vi "PMT_plus_Kiethley2450_plus_rotationstage.vi"() -> ()   [LabVIEW 2022 SP3]
uses:
  <vilib>/Analysis/1siggen.llb/Ramp Pattern by Delta.vi
  <vilib>/Utility/file.llb/Write Delimited Spreadsheet (string).vi
  <vilib>/Utility/file.llb/Write Delimited Spreadsheet (DBL).vi
  <vilib>/Analysis/NI_AALBase.lvlib
  C:/Users/Public/OneDrive/Desktop/test_save_lv22/Close.vi/Close Folder/Users/Public/OneDrive/Desktop/Keithley_2450_2470_1_4_0_LV2015_NewReadme2_2450-LV2015-1.4.0/Keithley 2450/Keithley 2450.lvlib
  C:/Users/Public/OneDrive/Desktop/PMT program/SampleCodeLabView/Kinesis_with_LabVIEW_Examples_LV12 - v3/Thorlabs.MotionControl.Controls.dll
  C:/Users/Public/OneDrive/Desktop/PMT program/SampleCodeLabView/Kinesis_with_LabVIEW_Examples_LV12 - v3/ThorLabs.MotionControl.KCube.DCServoCLI.dll
panel:
  in  "wait for move (ms)":u32=2000
  out "PC":dbl caption="Current Rotation Position"
  in  "quarter waveplate p2":dbl=221.0 format="%#_13g"
  in  "quarter waveplate p1":dbl=131.0 format="%#_13g"
  in  "Motor Controller\nSerialNumber":string="27268499"
  in  "KCubeDCServoControl":refnum<k24>(container)
  in  "Loop?":bool
  out "error out":errorcluster
  out "current 2450":dbl=2.5622937e-12 format="%e"
  out "Serial Configuration":T1={"Baud Rate"=9600, "Parity"=0, "Data Bits"=8, "Stop Bits"=10, "Flow Control"=0} {"Flow Control" items=["None", "XON/XOFF", "RTS/CTS", "XON/XOFF & RTS/CTS", "DTR/DSR", "XON/XOFF & DTR/DSR"]; "Stop Bits" items=["1.0"=10, "1.5"=15, "2.0"=20]; "Data Bits" items=["7"=7, "8"=8]; "Parity" items=["None", "Odd", "Even", "Mark", "Space"]; "Baud Rate" items=["300"=300, "600"=600, "1200"=1200, "2400"=2400, "4800"=4800, "9600"=9600, "19200"=19200]}
  in  "Use PMT?":bool=TRUE
  out "XY Graph":cluster{dbl[], dbl[]}(graph)={[-1.0, -0.5, 0.0], [45.5, 47.5, 49.0]}
  out "Actual Voltage 2450":dbl
  in  "Num Current Meas":i32=20
  in  "Path":path=path "C:/Users/Public/OneDrive/Desktop/test.txt"
  in  "error in (no error)":errorcluster
  in  "VISA resource name":refnum<visa-resource-name>="GPIB0::1::INSTR"
  out "Set Voltage 2450":dbl
  in  "Step Size (V)":dbl=0.5 format="%#_13g"
  in  "End V":dbl=-1.0 format="%#_13g"
  in  "Start V":dbl format="%#_13g"
  in  "Source Limit Level (0.1)":dbl=1e-08
  out "standard deviation":dbl
  out "mean":dbl=49.0
  out "data":u32[](array[numeric])=[49, 49]
  out "OLD":bool
  out "DB":u32[](array[numeric])=[49, 0, 0, 0, 0, 0, 0, 0, 0, 0, 0, 0, 0, 0, 0, 0]
  out "Overload":i32
  out "Gate Number":i32=1
  in  "Correction":bool=TRUE
  out "Num Gates Read":i32=2
  out "Gate Time Read":i32=100 caption="Gate time Read"
  out "Num Gates Set":i32=2
  out "Gate Time Set":i32=100
  out "PowerD":i32 caption="Power\nRead Data"
  out "Handle Number":i32=173123648
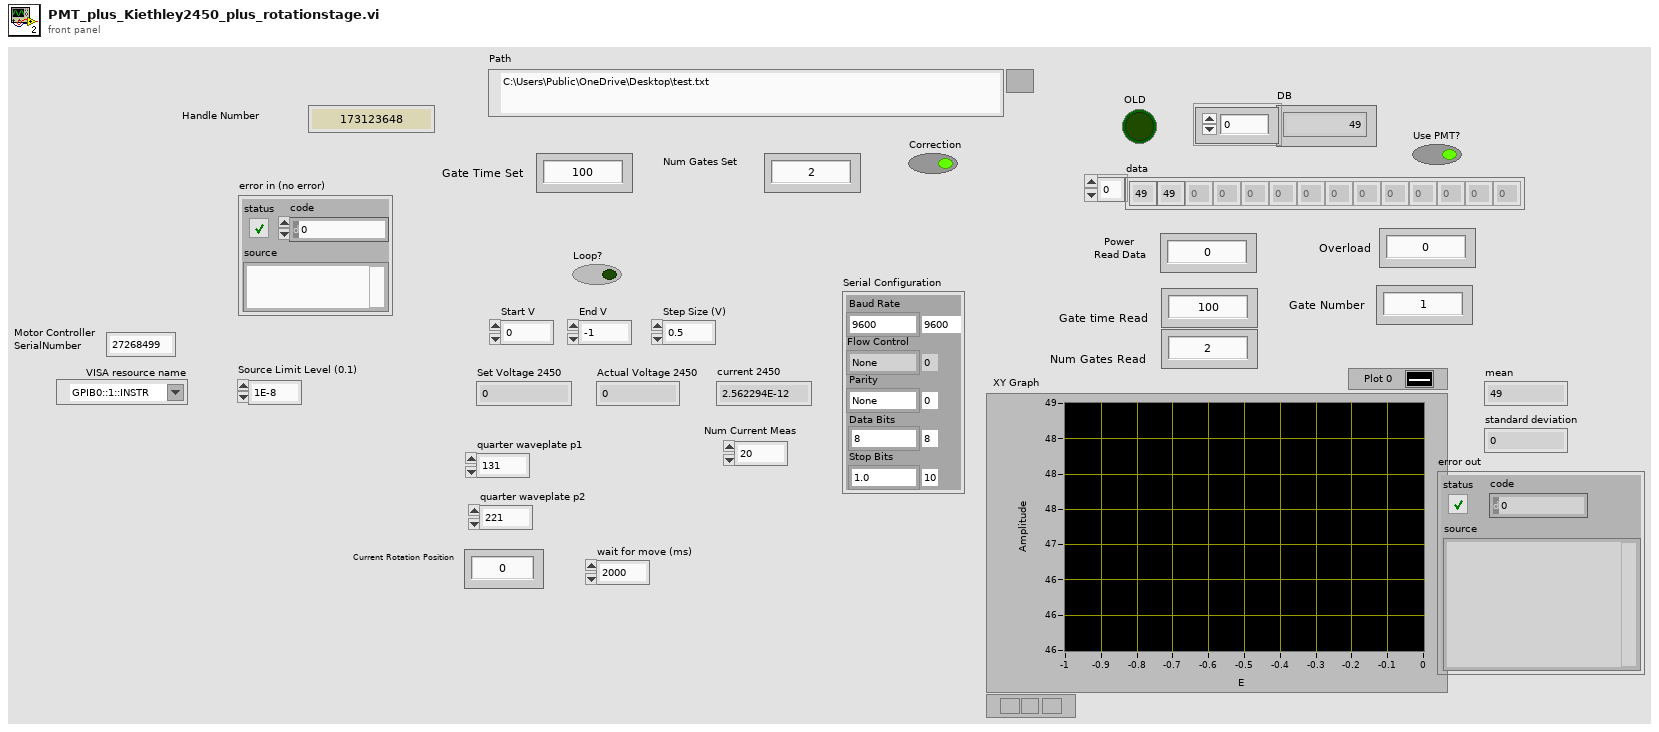
[diagram p1: front panel]
types:
  T1 = cluster{"Baud Rate":u32, "Parity":u16, "Data Bits":u16, "Stop Bits":u16, "Flow Control":u16}
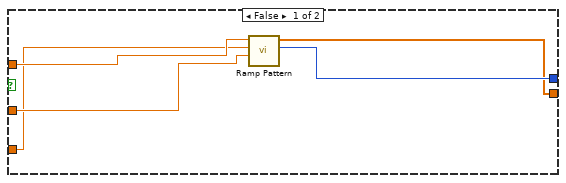
[diagram p2: hidden frame]
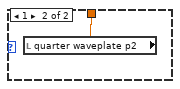
[diagram p3: hidden frame]
diagram:
  n1 = flat-sequence {
    tunnel: [w46] -> w20
    tunnel: [w37] -> w19
    tunnel: ["Path"] -> w18
    tunnel: [w36] -> w17
    tunnel: [w25] -> w16
    tunnel: [w22] -> w1
    tunnel: w20 -> [w82]
    tunnel: [w82] -> w15
    tunnel: w19 -> [w81]
    tunnel: [w81] -> w13
    tunnel: w18 -> [w80]
    tunnel: [w80] -> w11
    tunnel: w17 -> [w79]
    tunnel: [w79] -> w9
    tunnel: [w78] -> w7
    tunnel: w16 -> [w78]
    tunnel: ["wait for move (ms)"] -> w4
    tunnel: [w76] -> w2
    tunnel: w1 -> [w76]
    tunnel: w15 -> [w93]
    tunnel: [w93] -> w14
    tunnel: w13 -> [w92]
    tunnel: [w92] -> w12
    tunnel: w11 -> [w91]
    tunnel: [w91] -> w10
    tunnel: w9 -> [w90]
    tunnel: [w90] -> w8
    tunnel: w7 -> [w89]
    tunnel: [w88] -> w6
    tunnel: [w84] -> w5
    tunnel: w4 -> [w84]
    tunnel: [w83] -> w3
    tunnel: w2 -> [w83]
    tunnel: w14 -> [w105]
    tunnel: w12 -> [w104]
    tunnel: [w103] -> w21
    tunnel: w10 -> [w102]
    tunnel: w8 -> [w97]
    tunnel: w6 -> [w96]
    tunnel: w5 -> [w95]
    tunnel: w3 -> [w94]
    tunnel: w21 -> [w570]
    frame #0 {
      # "open PMT and turn on power"
      n2 = local write "quarter waveplate p2"("quarter waveplate p2") -> ()
      n3 = local write "quarter waveplate p1"("quarter waveplate p1") -> ()
      n4 = call "Open.vi"("Serial Number"="30430219") -> ("Handle Number"=w50:i32)  [unwired: 9 in, 1 out]
      "Handle Number" <- w50
      n5 = case shown="True" "Loop?" {
        tunnel: "Start V" -> [w57 w68]
        tunnel: "End V" -> [w56 w66]
        tunnel: [w59 w65] -> w36
        tunnel: [w60 w64] -> w37
        tunnel: "Step Size (V)" -> [w58 w62]
        frame False {
          n6 = call-poly <vilib>:"Ramp Pattern.vi"("start"=w57, "end"=w56, "delta"=w58) -> ("samples"=w60:i32, "Ramp Pattern"=w59:dbl[])  [unwired: 6 in, 1 out]
        }
        frame True {
          w63 = -1.0
          n7 = Multiply(x=w62, y=w63) -> (x*y=w61:dbl)
          n8 = Multiply(x=w66, y=w63) -> (x*y=w67:dbl)
          n9 = call-poly <vilib>:"Ramp Pattern.vi"("start"=w68, "end"=w66, "delta"=w62) -> ("samples"=w72:i32, "Ramp Pattern"=w69:dbl[])  [unwired: 6 in, 1 out]
          n10 = call-poly <vilib>:"Ramp Pattern.vi"("start"=w67, "end"=w68, "delta"=w62) -> ("samples"=w75:i32, "Ramp Pattern"=w71:dbl[])  [unwired: 6 in, 1 out]
          n11 = call-poly <vilib>:"Ramp Pattern.vi"("start"=w66, "end"=w67, "delta"=w61) -> ("samples"=w73:i32, "Ramp Pattern"=w70:dbl[])  [unwired: 6 in, 1 out]
          n12 = Add(x=w72, y=w73) -> (x+y=w74:i32)
          n13 = Build Array (concatenate)(w69, w70, w71) -> (w65:dbl[])
          n14 = Add(x=w74, y=w75) -> (x+y=w64:i32)
        }
      }
      n15 = call "Read HV.vi"("handle"=w50) -> ("HV out"=w49:i32, "handle out"=w53:i32)  [unwired: 8 in, 1 out]
      n16 = Boolean To (0,1)(Boolean="Use PMT?") -> (0, 1=w51:i16)
      n17 = local write "PowerD"(w49) -> ()
      n18 = To Long Integer(number=w51) -> (32bit integer=w52:i32)
      n19 = call "Set HV.vi"("HV"=w52, "handle"=w53) -> ("handle out"=w55:i32)  [unwired: 8 in, 1 out]
      n20 = property class="KCubeDCServoControl"(reference="KCubeDCServoControl", "SerialNumber"="Motor Controller\nSerialNumber") -> (reference out=w35:refnum<k24>)  [unwired: 1 in, 1 out]
      n21 = invoke class="KCubeDCServoControl" method="CreateDevice"(reference=w35) -> (reference out=w32:refnum<k24>)  [unwired: 2 in, 2 out]
      n22 = property class="KCubeDCServoControl"(reference=w32) -> ("Device"=w22:refnum<k24>)  [unwired: 1 in, 2 out]
      n23 = call "Read HV.vi"("handle"=w55) -> ("HV out"=w54:i32, "handle out"=w46:i32)  [unwired: 8 in, 1 out]
      n24 = local write "PowerD"(w54) -> ()
      n25 = invoke class="KCubeDCServo" method="GetPositionCounter"(reference=w22) -> (reference out=w28:refnum<k24>, "GetPositionCounter"=w31:i32)  [unwired: 2 in, 1 out]
      n26 = Divide(x=w31, y=1919.6418578623338) -> (x/y=w29:dbl)
      n27 = local write "PC"(w29) -> ()
      n28 = invoke class="KCubeDCServo" method="SetMoveAbsolutePosition"(reference=w28, "position"="quarter waveplate p1") -> (reference out=w27:refnum<k24>)  [unwired: 2 in, 3 out]
      n29 = invoke class="KCubeDCServo" method="MoveAbsolute"(reference=w27, "waitTimeout"=0) -> (reference out=w25:refnum<k24>)  [unwired: 2 in, 3 out]
      n30 = Build Array("# SetVoltage2450(V) ActualVoltage2450(V) CountsMean CountsStd Current2450(uA) Current2450Std(uA)") -> (w41:string[])
      n31 = call-poly <vilib>:"Write Delimited Spreadsheet.vi"("file path (dialog if empty)"="Path", "1D data"=w41, "append to file? (new file:F)"=TRUE) -> ()  [unwired: 11 in, 2 out]
    }
    frame #1 {
      n32 = Wait (ms)(milliseconds to wait="wait for move (ms)") -> ()  [unwired: 1 out]
    }
    frame #2 {
      n33 = invoke class="KCubeDCServo" method="GetPositionCounter"(reference=w89) -> (reference out=w88:refnum<k24>, "GetPositionCounter"=w86:i32)  [unwired: 2 in, 1 out]
      n34 = Divide(x=w86, y=1919.6418578623338) -> (x/y=w85:dbl)
      n35 = local write "PC"(w85) -> ()
    }
    frame #3 {
      w100 = 0
      w101 = 0
      n36 = Initialize Array(w101, w101) -> (w98:i32[])
      n37 = Initialize Array(w100, w100) -> (w99:i32[])
      n38 = for {
        N: w104 -> [_]
        tunnel: w97 -> [w159] mode=indexing
        tunnel: w105 -> [w135]
        tunnel: [w158] -> w103
        tunnel: w102 -> [w131]
        shift-right: [w149] -> _
        shift-left: w98 -> [w154]
        shift-right: [w150] -> _
        shift-left: w99 -> [w153]
        tunnel: w96 -> [w127]
        tunnel: w95 -> [w123]
        tunnel: w94 -> [w109]
        n39 = flat-sequence {
          tunnel: w153 -> [w193]
          tunnel: w154 -> [w194]
          tunnel: w159 -> [w185]
          tunnel: [w185] -> w148
          tunnel: [w194] -> w146
          tunnel: [w193] -> w144
          tunnel: [w189] -> w142
          tunnel: [w188] -> w140
          tunnel: ["Num Current Meas"] -> w136
          tunnel: w135 -> [w163]
          tunnel: [w163] -> w132
          tunnel: w131 -> [w162]
          tunnel: [w162] -> w128
          tunnel: w127 -> [w161]
          tunnel: [w161] -> w124
          tunnel: w109 -> [w160]
          tunnel: [w160] -> w107
          tunnel: w148 -> [w205]
          tunnel: [w205] -> w147
          tunnel: w146 -> [w204]
          tunnel: [w204] -> w145
          tunnel: w144 -> [w203]
          tunnel: [w203] -> w143
          tunnel: w142 -> [w202]
          tunnel: [w202] -> w141
          tunnel: w140 -> [w201]
          tunnel: [w201] -> w139
          tunnel: [w200] -> w137
          tunnel: w136 -> [w200]
          tunnel: [w198] -> w133
          tunnel: w132 -> [w198]
          tunnel: [w197] -> w129
          tunnel: w128 -> [w197]
          tunnel: [w196] -> w125
          tunnel: w124 -> [w196]
          tunnel: [w195] -> w108
          tunnel: w107 -> [w195]
          tunnel: [w236] -> w157
          tunnel: [w237] -> w156
          tunnel: [w229] -> w155
          tunnel: [w235] -> w152
          tunnel: [w234] -> w151
          tunnel: w147 -> [w236]
          tunnel: w145 -> [w235]
          tunnel: w143 -> [w234]
          tunnel: w141 -> [w232]
          tunnel: w139 -> [w233]
          tunnel: [w230] -> w138
          tunnel: w137 -> [w231]
          tunnel: [w209] -> w134
          tunnel: w133 -> [w209]
          tunnel: [w208] -> w130
          tunnel: w129 -> [w208]
          tunnel: [w207] -> w126
          tunnel: w125 -> [w207]
          tunnel: w108 -> [w206]
          tunnel: [w206] -> w106
          tunnel: w157 -> [w261]
          tunnel: w156 -> [w260]
          tunnel: w155 -> [w259]
          tunnel: w152 -> [w258]
          tunnel: w151 -> [w257]
          tunnel: [w262] -> w122
          tunnel: [w256] -> w119
          tunnel: w138 -> [w255]
          tunnel: w134 -> [w254]
          tunnel: w130 -> [w250]
          tunnel: w126 -> [w252]
          tunnel: w123 -> [w251]
          tunnel: [w250] -> w117
          tunnel: [w249] -> w116
          tunnel: [w244] -> w115
          tunnel: [w243] -> w114
          tunnel: [w242] -> w113
          tunnel: [w241] -> w112
          tunnel: [w240] -> w111
          tunnel: [w239] -> w110
          tunnel: w106 -> [w238]
          tunnel: w122 -> [w565]
          tunnel: [w565] -> w121
          tunnel: [w553] -> w120
          tunnel: w119 -> [w564]
          tunnel: [w564] -> w118
          tunnel: w117 -> [w562]
          tunnel: w116 -> [w560]
          tunnel: w115 -> [w559]
          tunnel: w114 -> [w558]
          tunnel: w113 -> [w557]
          tunnel: w112 -> [w556]
          tunnel: w111 -> [w554]
          tunnel: w110 -> [w552]
          tunnel: [w567] -> w149
          tunnel: [w568] -> w150
          tunnel: [w569] -> w158
          tunnel: w121 -> [w569]
          tunnel: w120 -> [w568]
          tunnel: w118 -> [w567]
          frame #0 {
            w172 = 1
            w174 = 0
            w183 = TRUE
            n40 = call "Initialize.vi"("error in (no error)"="error in (no error)", "Reset (True)"=FALSE, "ID Query (True)"=TRUE, "VISA resource name"="VISA resource name") -> ("error out"=w170:errorcluster, "VISA resource name out"=w171:refnum<visa-resource-name>)  [unwired: 6 in]
            n41 = call "Clear Buffer.vi"("VISA resource name"=w171, "error in (no error)"=w170) -> ("VISA resource name out"=w168:refnum<visa-resource-name>, "error out"=w169:errorcluster)  [unwired: 12 in]
            n42 = call "Configure Measurement Range.vi"("error in (no error)"=w169, "Enable Auto Range (T:Enable)"=w183, "Function (0: Volts)"=w174, "VISA resource name"=w168) -> ("error out"=w182:errorcluster, "VISA resource name out"=w181:refnum<visa-resource-name>)  [unwired: 6 in]
            n43 = call "Configure Measurement Range.vi"("error in (no error)"=w182, "Enable Auto Range (T:Enable)"=w183, "Function (0: Volts)"=w172, "VISA resource name"=w181) -> ("error out"=w178:errorcluster, "VISA resource name out"=w175:refnum<visa-resource-name>)  [unwired: 6 in]
            n44 = call "Configure Output.vi"("VISA resource name"=w175, "Source Level (0)"=w185, "Source Limit Level (0.1)"="Source Limit Level (0.1)", "error in (no error)"=w178) -> ("VISA resource name out"=w176:refnum<visa-resource-name>, "error out"=w179:errorcluster)  [unwired: 10 in]
            n45 = call "Configure Source Function.vi"("error in (no error)"=w179, "Function (0: Volts)"=w174, "VISA resource name"=w176) -> ("error out"=w180:errorcluster, "VISA resource name out"=w177:refnum<visa-resource-name>)  [unwired: 7 in]
            n46 = call "Configure Measurement Function.vi"("error in (no error)"=w180, "Function (0: Volts)"=w172, "VISA resource name"=w177) -> ("error out"=w164:errorcluster, "VISA resource name out"=w167:refnum<visa-resource-name>)  [unwired: 7 in]
            n47 = call "Set Measurement Count.vi"("error in (no error)"=w164, "Measurement Count (1)"="Num Current Meas", "VISA resource name"=w167) -> ("error out"=w165:errorcluster, "VISA resource name out"=w166:refnum<visa-resource-name>)  [unwired: 7 in]
            n48 = call "Enable Output.vi"("error in (no error)"=w165, "Enable Output (T: Enable)"=TRUE, "VISA resource name"=w166) -> ("error out"=w189:errorcluster, "VISA resource name out"=w188:refnum<visa-resource-name>)  [unwired: 7 in]
            "Set Voltage 2450" <- w185
          }
          frame #1 {
            n49 = Wait (ms)(milliseconds to wait=u32 100) -> ()  [unwired: 1 out]
          }
          frame #2 {
            w213 = 1000000
            n50 = call "Make Reading and Store in Buffer.vi"("VISA resource name"=w233, "error in (no error)"=w232) -> ("VISA resource name out"=w225:refnum<visa-resource-name>, "error out"=w224:errorcluster)  [unwired: 12 in]
            n51 = call "Read (Multiple Points).vi"("VISA resource name"=w225, "Start Index (1)"=u32 1, "End Index (1)"=w231, "error in (no error)"=w224) -> ("VISA resource name out"=w217:refnum<visa-resource-name>, "Data out"=w222:string, "error out"=w216:errorcluster)  [unwired: 9 in]
            n52 = call "Get Source Level.vi"("error in (no error)"=w216, "VISA resource name"=w217) -> ("error out"=w227:errorcluster, "Voltage Level Out"=w237:dbl, "VISA resource name out"=w228:refnum<visa-resource-name>)  [unwired: 6 in, 1 out]
            "Actual Voltage 2450" <- w237
            n53 = Spreadsheet String To Array(delimiter (Tab)=",", format string="%s", spreadsheet string=w222, array type (2D Dbl)=dbl[] []) -> (array=w218:dbl[])
            n54 = call "Enable Output.vi"("error in (no error)"=w227, "Enable Output (T: Enable)"=TRUE, "VISA resource name"=w228) -> ("error out"=w210:errorcluster, "VISA resource name out"=w211:refnum<visa-resource-name>)  [unwired: 7 in]
            n55 = call "Close.vi"("error in (no error)"=w210, "VISA resource name"=w211) -> ("error out"=→"error out":errorcluster)  [unwired: 9 in]
            n56 = call <vilib>:"Std Deviation and Variance.vi"("X"=w218) -> ("mean"=w214:dbl, "standard deviation"=w215:dbl)  [unwired: 1 in, 1 out]
            "current 2450" <- w214
            n57 = Multiply(x=w215, y=w213) -> (x*y=w230:dbl)
            n58 = Multiply(x=w214, y=w213) -> (x*y=w229:dbl)
          }
          frame #3 {
            w246 = 0
            w248 = 0
            n59 = Initialize Array(w248, w248) -> (w247:i32[])
            n60 = Initialize Array(w246, w246) -> (w245:i32[])
            n61 = for {
              N: 2 -> [_]
              tunnel: w261 -> [w371]
              tunnel: w260 -> [w370]
              tunnel: w259 -> [w369]
              tunnel: w258 -> [w291] mode=indexing
              tunnel: w257 -> [w368] mode=indexing
              tunnel: [w367] -> w256
              tunnel: w255 -> [w366]
              shift-right: [w372] -> w262
              shift-left: w254 -> [w365]
              tunnel: w252 -> [w303]
              tunnel: w251 -> [w302]
              tunnel: [w292] -> w249
              shift-right: [w270] -> w244
              shift-left: w247 -> [w290]
              shift-right: [w269] -> w243
              shift-left: w245 -> [w280]
              tunnel: [w268] -> w242
              tunnel: [w267] -> w241
              tunnel: [w266] -> w240
              tunnel: [w265] -> w239
              tunnel: w238 -> [w264]
              i -> [w301]
              (unwired) "# SetVoltage2450(V) ActualVoltage2450(V) CountsMean CountsStd Current2450(uA) Current2450Std(uA)"
              # "- actual voltage array\n- actual voltage current\n- set voltage current\n-  current current\n- current std current"
              n62 = flat-sequence {
                tunnel: [w384] -> w317
                tunnel: [w382] -> w315
                tunnel: [w383] -> w313
                tunnel: w371 -> [w384]
                tunnel: w370 -> [w383]
                tunnel: w369 -> [w382]
                tunnel: w291 -> [w381]
                tunnel: [w381] -> w311
                tunnel: w368 -> [w380]
                tunnel: [w380] -> w309
                tunnel: w366 -> [w379]
                tunnel: [w379] -> w307
                tunnel: w365 -> [w378]
                tunnel: [w378] -> w305
                tunnel: w303 -> [_]
                tunnel: w301 -> [w376]
                tunnel: w290 -> [w375]
                tunnel: [w375] -> w286
                tunnel: w280 -> [w374]
                tunnel: [w374] -> w273
                tunnel: w264 -> [w373]
                tunnel: [w373] -> w263
                tunnel: w317 -> [w397]
                tunnel: [w397] -> w316
                tunnel: w315 -> [w396]
                tunnel: [w396] -> w314
                tunnel: w313 -> [w395]
                tunnel: [w395] -> w312
                tunnel: w311 -> [w394]
                tunnel: [w394] -> w310
                tunnel: w309 -> [w393]
                tunnel: [w393] -> w308
                tunnel: w307 -> [w392]
                tunnel: [w392] -> w306
                tunnel: w305 -> [w391]
                tunnel: [w391] -> w304
                tunnel: [w389] -> w287
                tunnel: w286 -> [w389]
                tunnel: [w388] -> w274
                tunnel: w273 -> [w388]
                tunnel: w263 -> [w387]
                tunnel: [w401] -> w364
                tunnel: [w407] -> w363
                tunnel: w316 -> [w407]
                tunnel: [w406] -> w362
                tunnel: w314 -> [w406]
                tunnel: [w405] -> w361
                tunnel: w312 -> [w405]
                tunnel: [w404] -> w360
                tunnel: w310 -> [w404]
                tunnel: [w403] -> w359
                tunnel: w308 -> [w403]
                tunnel: [w402] -> w358
                tunnel: w306 -> [w402]
                tunnel: w304 -> [w401]
                tunnel: w302 -> [w400]
                tunnel: [w399] -> w288
                tunnel: w287 -> [w399]
                tunnel: [w398] -> w275
                tunnel: w274 -> [w398]
                tunnel: w364 -> [w422]
                tunnel: [w417] -> w357
                tunnel: [w415] -> w356
                tunnel: w363 -> [w415]
                tunnel: [w414] -> w355
                tunnel: w362 -> [w414]
                tunnel: [w413] -> w354
                tunnel: w361 -> [w413]
                tunnel: [w412] -> w353
                tunnel: w360 -> [w412]
                tunnel: [w411] -> w352
                tunnel: w359 -> [w411]
                tunnel: [w410] -> w351
                tunnel: w358 -> [w410]
                tunnel: [w409] -> w289
                tunnel: w288 -> [w409]
                tunnel: [w408] -> w276
                tunnel: w275 -> [w408]
                tunnel: [w433] -> w350
                tunnel: w357 -> [w435]
                tunnel: [w430] -> w349
                tunnel: w356 -> [w430]
                tunnel: w355 -> [w429]
                tunnel: [w429] -> w348
                tunnel: [w428] -> w347
                tunnel: w354 -> [w428]
                tunnel: [w427] -> w346
                tunnel: w353 -> [w427]
                tunnel: [w426] -> w345
                tunnel: w352 -> [w426]
                tunnel: [w425] -> w344
                tunnel: w351 -> [w425]
                tunnel: w289 -> [w424]
                tunnel: [w424] -> w283
                tunnel: [w423] -> w277
                tunnel: w276 -> [w423]
                tunnel: w350 -> [w450]
                tunnel: [w450] -> w343
                tunnel: [w446] -> w342
                tunnel: [w446] -> w341
                tunnel: [w445] -> w340
                tunnel: w349 -> [w445]
                tunnel: [w444] -> w339
                tunnel: w348 -> [w444]
                tunnel: w347 -> [w443]
                tunnel: [w443] -> w338
                tunnel: [w442] -> w337
                tunnel: w346 -> [w442]
                tunnel: [w441] -> w336
                tunnel: w345 -> [w441]
                tunnel: w344 -> [w440]
                tunnel: [w440] -> w335
                tunnel: [w439] -> w284
                tunnel: w283 -> [w439]
                tunnel: [w438] -> w278
                tunnel: w277 -> [w438]
                tunnel: w343 -> [w465]
                tunnel: [w461] -> w334
                tunnel: w342 -> [w460]
                tunnel: w341 -> [w459]
                tunnel: [w460] -> w333
                tunnel: [w459] -> w332
                tunnel: w340 -> [w458]
                tunnel: [w458] -> w331
                tunnel: [w457] -> w330
                tunnel: w339 -> [w457]
                tunnel: [w456] -> w329
                tunnel: w338 -> [w456]
                tunnel: [w455] -> w328
                tunnel: w337 -> [w455]
                tunnel: [w454] -> w327
                tunnel: w336 -> [w454]
                tunnel: [w453] -> w326
                tunnel: w335 -> [w453]
                tunnel: [w452] -> w285
                tunnel: w284 -> [w452]
                tunnel: [w451] -> w279
                tunnel: w278 -> [w451]
                tunnel: [w480] -> w325
                tunnel: w334 -> [w479]
                tunnel: w333 -> [w478]
                tunnel: w332 -> [w477]
                tunnel: [w476] -> w324
                tunnel: [w473] -> w323
                tunnel: w331 -> [w473]
                tunnel: [w472] -> w322
                tunnel: w330 -> [w472]
                tunnel: w329 -> [w471]
                tunnel: [w471] -> w321
                tunnel: [w470] -> w320
                tunnel: w328 -> [w470]
                tunnel: [w469] -> w319
                tunnel: w327 -> [w469]
                tunnel: [w468] -> w318
                tunnel: w326 -> [w468]
                tunnel: w285 -> [w467]
                tunnel: [w467] -> w282
                tunnel: w279 -> [w466]
                tunnel: [w466] -> w272
                tunnel: w325 -> [w536]
                tunnel: [w535] -> w299
                tunnel: [w534] -> w300
                tunnel: w324 -> [w534]
                tunnel: w323 -> [w533]
                tunnel: [w533] -> w298
                tunnel: [w532] -> w297
                tunnel: w322 -> [w532]
                tunnel: [w531] -> w296
                tunnel: w321 -> [w531]
                tunnel: [w530] -> w295
                tunnel: w320 -> [w530]
                tunnel: w319 -> [w529]
                tunnel: [w529] -> w294
                tunnel: [w528] -> w293
                tunnel: w318 -> [w528]
                tunnel: w282 -> [w527]
                tunnel: [w527] -> w281
                tunnel: w272 -> [w526]
                tunnel: [w526] -> w271
                tunnel: [w551] -> w372
                tunnel: w299 -> [w551]
                tunnel: w298 -> [w547]
                tunnel: w297 -> [w541]
                tunnel: w296 -> [w539]
                tunnel: w295 -> [w550]
                tunnel: w294 -> [w540]
                tunnel: [w549] -> w367
                tunnel: w293 -> [w538]
                tunnel: w300 -> [w548]
                tunnel: [w547] -> w292
                tunnel: w281 -> [w546]
                tunnel: w271 -> [w545]
                tunnel: [w543] -> w270
                tunnel: [w542] -> w269
                tunnel: [w541] -> w268
                tunnel: [w538] -> w267
                tunnel: [w540] -> w266
                tunnel: [w539] -> w265
                frame #0 {
                  n63 = case shown="0, Default" w376 {
                    tunnel: [w385 w386] -> w377
                    frame 0, Default {
                      n64 = local read "quarter waveplate p1"() -> (w385:dbl)
                    }
                    frame 1 {
                      n65 = local read "quarter waveplate p2"() -> (w386:dbl)
                    }
                  }
                  n66 = invoke class="KCubeDCServo" method="SetMoveAbsolutePosition"(reference=w373, "position"=w377) -> ()  [unwired: 2 in, 4 out]
                }
                frame #1 {
                  n67 = invoke class="KCubeDCServo" method="MoveAbsolute"(reference=w387, "waitTimeout"=0) -> ()  [unwired: 2 in, 4 out]
                }
                frame #2 {
                  n68 = Wait (ms)(milliseconds to wait=w400) -> ()  [unwired: 1 out]
                }
                frame #3 {
                  # "set gate time"
                  n69 = local read "Gate Time Set"() -> (w419:i32)
                  n70 = Wait (ms)(milliseconds to wait=u32 200) -> ()  [unwired: 1 out]
                  n71 = To Long Integer(number=w419) -> (32bit integer=w420:i32)
                  n72 = call "Set IT.vi"("IT"=w420, "handle"=w422) -> ("handle out"=w421:i32)  [unwired: 8 in, 1 out]
                  n73 = call "Read IT.vi"("handle"=w421) -> ("IT out"=w418:i32, "handle out"=w417:i32)  [unwired: 8 in, 1 out]
                  n74 = local write "Gate Time Read"(w418) -> ()
                }
                frame #4 {
                  # "set number of gates"
                  n75 = local read "Num Gates Set"() -> (w437:i32)
                  n76 = Wait (ms)(milliseconds to wait=u32 200) -> ()  [unwired: 1 out]
                  n77 = To Long Integer(number=w437) -> (32bit integer=w436:i32)
                  n78 = call "Set RN.vi"("RN"=w436, "handle"=w435) -> ("handle out"=w434:i32)  [unwired: 8 in, 1 out]
                  n79 = call "Read RN.vi"("handle"=w434) -> ("RN out"=w432:i32, "handle out"=w433:i32)  [unwired: 8 in, 1 out]
                  n80 = local write "Num Gates Read"(w432) -> ()
                }
                frame #5 {
                  # "gate number data"
                  # "count data"
                  n81 = local write "Gate Number"(0) -> ()
                  n82 = Initialize Array(u32 0, 0 ("次元サイズ")) -> (w446:u32[])
                }
                frame #6 {
                  n83 = Boolean To (0,1)(Boolean="Correction") -> (0, 1=w464:i16)
                  n84 = To Long Integer(number=w464) -> (32bit integer=w463:i32)
                  n85 = call "Count Start.vi"("Correction"=w463, "handle"=w465) -> ("handle out"=w461:i32)  [unwired: 8 in, 1 out]
                }
                frame #7 {
                  n86 = local read "Num Gates Read"() -> (w475:i32)
                  n87 = for {
                    N: w475 -> [_]
                    shift-right: [w481] -> w476
                    shift-left: w478 -> [w489]
                    shift-right: [w485] -> _
                    shift-left: w477 -> [w488]
                    tunnel: w479 -> [w490]
                    tunnel: [w491] -> w480
                    tunnel: [w481] -> w474
                    n88 = flat-sequence {
                      tunnel: [w501] -> w495
                      tunnel: [w500] -> w486
                      tunnel: [w499] -> w483
                      tunnel: w490 -> [w501]
                      tunnel: w489 -> [w500]
                      tunnel: w488 -> [w499]
                      tunnel: [w512] -> w494
                      tunnel: w495 -> [w511]
                      tunnel: [w506] -> w493
                      tunnel: [w505] -> w492
                      tunnel: [w504] -> w487
                      tunnel: w486 -> [w504]
                      tunnel: [w503] -> w484
                      tunnel: w483 -> [w503]
                      tunnel: [w502] -> w482
                      tunnel: w494 -> [w525]
                      tunnel: w493 -> [w520]
                      tunnel: w492 -> [w519]
                      tunnel: w487 -> [w517]
                      tunnel: w484 -> [w516]
                      tunnel: w482 -> [w515]
                      tunnel: [w525] -> w491
                      tunnel: [w518] -> w481
                      tunnel: [w513] -> w485
                      frame #0 {
                        n89 = Initialize Array(u32 0, 16 ("次元サイズ")) -> (w496:u32[])
                        n90 = local write "DB"(w496) -> ()
                      }
                      frame #1 {
                        # "read data"
                        n91 = local read "Gate Number"() -> (w510:i32)
                        n92 = local read "Overload"() -> (w509:i32)
                        n93 = local read "DB"() -> (w507:u32[])
                        n94 = call "Read Data.vi"("OLD"=w509, "DataBuf"=w507, "GateNum"=w510, "handle"=w511) -> ("OLD out"=w508:i32, "DataBuf out"=w505:u32[], "GateNum out"=w502:i32, "handle out"=w512:i32, "function return"=w506:u32)  [unwired: 3 in]
                        n95 = local write "Gate Number"(w502) -> ()
                        n96 = local write "DB"(w505) -> ()
                        n97 = local write "Overload"(w508) -> ()
                      }
                      frame #2 {
                        # "Pickup Tans Data!"
                        n98 = To Long Integer(number=w520) -> (32bit integer=w521:i32)
                        n99 = Build Array(w515) -> (w514:i32[])
                        n100 = local read "Overload"() -> (w523:i32)
                        n101 = Build Array (concatenate)(w516, w514) -> (w513:u32[])
                        n102 = Array Subset(array=w519, length=w521) -> (w522:u32[])  [unwired: 1 in]
                        n103 = Not Equal To 0?(x=w523) -> (x != 0?=→"OLD":bool)
                        n104 = Build Array (concatenate)(w517, w522) -> (w518:u32[])
                      }
                    }
                  }
                  "data" <- w474
                }
                frame #8 {
                  # "data"
                  n105 = call "Count Stop.vi"("handle"=w536) -> ("handle out"=w535:i32)  [unwired: 9 in, 1 out]
                }
                frame #9 {
                  n106 = call <vilib>:"Std Deviation and Variance.vi"("X"=w548) -> ("mean"=w537:dbl, "standard deviation"=w544:dbl)  [unwired: 1 in, 1 out]
                  "mean" <- w537
                  "standard deviation" <- w544
                  n107 = Build Array (concatenate)(w545, w544) -> (w542:dbl[])
                  n108 = Build Array (concatenate)(w546, w537) -> (w543:dbl[])
                  n109 = Build Array(w550, w537) -> (w549:dbl[])
                }
              }
            }
          }
          frame #4 {
            (unwired) "# SetVoltage2450(V) ActualVoltage2450(V) CountsMeanCirc1 CountsMeanCirc2 CountsStdCirc1 CountsStdCirc2 Current2450(uA) Current2450Std(uA)"
            n110 = Build Array(w554, w552) -> (w553:dbl[])
            n111 = Build Array (concatenate)(w560, w552, w559, w558, w557, w556) -> (w555:dbl[])
            n112 = call-poly <vilib>:"Write Delimited Spreadsheet.vi"("file path (dialog if empty)"=w562, "format (%.3f)"="%.10f", "1D data"=w555, "append to file? (new file:F)"=TRUE) -> ()  [unwired: 10 in, 2 out]
          }
          frame #5 {
            n113 = Bundle(w568, w567) -> (→"XY Graph":cluster{dbl[], dbl[]})  [unwired: 1 in]
          }
        }
      }
    }
    frame #4 {
      # "turn off PMT and close"
      n114 = Boolean To (0,1)(Boolean=FALSE) -> (0, 1=w575:i16)
      n115 = To Long Integer(number=w575) -> (32bit integer=w574:i32)
      n116 = call "Set HV.vi"("HV"=w574, "handle"=w570) -> ("handle out"=w572:i32)  [unwired: 8 in, 1 out]
      n117 = call "Read HV.vi"("handle"=w572) -> ("HV out"=w576:i32, "handle out"=w571:i32)  [unwired: 8 in, 1 out]
      n118 = call "Close.vi"("Handle"=w571) -> ()  [unwired: 9 in, 2 out]
      n119 = local write "PowerD"(w576) -> ()
    }
  }
